vi "PhotonPipelineResult_Equals.vi"(9 "Other PhotonPipelineResult":T1 {"Targets"."CameraToTarget"."ROTATION"."SIN" format="%13.4f"; "Targets"."CameraToTarget"."ROTATION"."COS" format="%13.4f"; "Targets"."CameraToTarget"."ROTATION"."VALUE" format="%13.4f"; "Targets"."CameraToTarget"."TRANSLATION"."Y" format="%14.3f"; "Targets"."CameraToTarget"."TRANSLATION"."X" format="%14.3f"}, 11 "PhotonPipelineResult":T1 {"Targets"."CameraToTarget"."ROTATION"."SIN" format="%13.4f"; "Targets"."CameraToTarget"."ROTATION"."COS" format="%13.4f"; "Targets"."CameraToTarget"."ROTATION"."VALUE" format="%13.4f"; "Targets"."CameraToTarget"."TRANSLATION"."Y" format="%14.3f"; "Targets"."CameraToTarget"."TRANSLATION"."X" format="%14.3f"}) -> (3 "Equal":bool)   [LabVIEW 2019, in "PhotonVisionLib.lvlib"]
doc: "Determines if two PipelineResults are equal.\n\nInputs:\n - PipelineResult -- PipelineResult cluster.\n - Other PipelineResult -- Other PipelineResult cluster.\n\nOutputs:\n - Equal -- Returns TRUE, if both pipeline results are equal.."
uses:
  PhotonVisionLib.lvlib
  TypeDef/PhotonPipelineResultType.ctl
  TypeDef/PhotonTrackedTargetType.ctl
  TypeDef/TargetCornerType.ctl
  <vilib>/Rock Robotics/WPI/ThirdParty/JAS_Junk/TrajLib/TRANSFORM2D.ctl
  <vilib>/Rock Robotics/WPI/ThirdParty/JAS_Junk/TrajLib/TRANSLATION2D.ctl
  <vilib>/Rock Robotics/WPI/ThirdParty/JAS_Junk/TrajLib/ROTATION2D.ctl
  <vilib>/Rock Robotics/WPI/ThirdParty/JAS_Junk/TrajLib/Trajectory_Library.lvlib
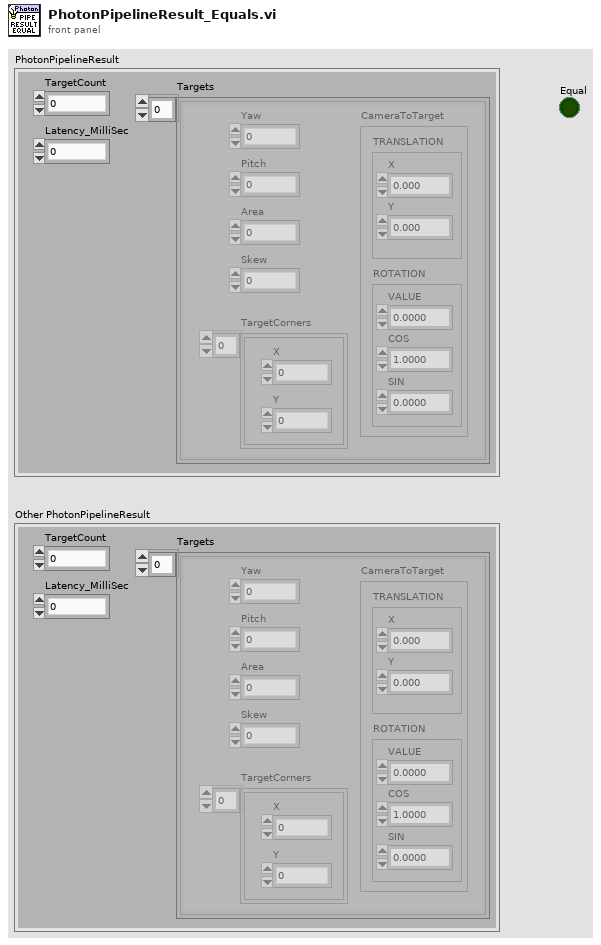
[diagram p1: front panel]
types:
  T1 = typedef "PhotonVisionLib.lvlib/PhotonPipelineResultType.ctl" = cluster{"TargetCount":i32, "Latency_MilliSec":dbl, "Targets":T2[]}
  T2 = typedef "PhotonVisionLib.lvlib/PhotonTrackedTargetType.ctl" = cluster{"Yaw":dbl, "Pitch":dbl, "Area":dbl, "Skew":dbl, "TargetCorners":T3[], "CameraToTarget":T4}
  T3 = typedef "PhotonVisionLib.lvlib/TargetCornerType.ctl" = cluster{"X":dbl, "Y":dbl}
  T4 = typedef "Trajectory_Library.lvlib/TRANSFORM2D.ctl" = cluster{"TRANSLATION":T5, "ROTATION":T6}
  T5 = typedef "Trajectory_Library.lvlib/TRANSLATION2D.ctl" = cluster{"X":dbl, "Y":dbl}
  T6 = typedef "Trajectory_Library.lvlib/ROTATION2D.ctl" = cluster{"VALUE":dbl, "COS":dbl, "SIN":dbl}
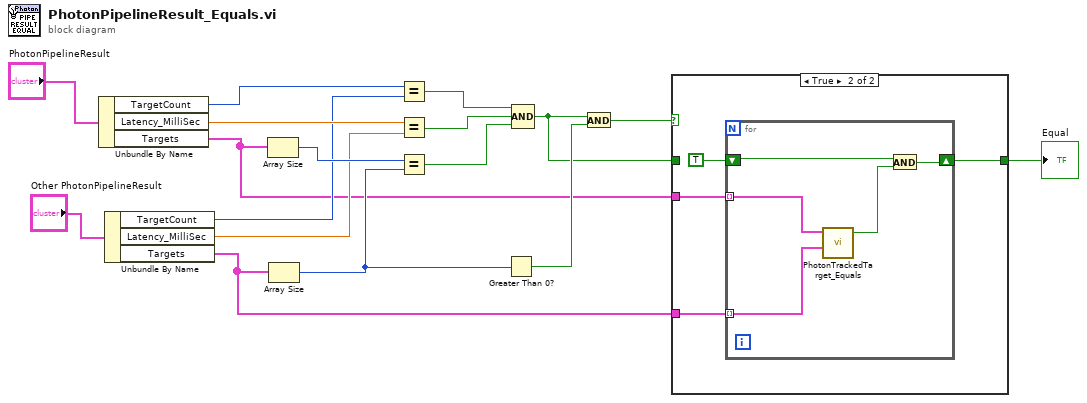
[diagram p0: block diagram]
diagram:
  n1 = Unbundle By Name("PhotonPipelineResult") -> ("TargetCount"=w15:i32, "Latency_MilliSec"=w14:dbl, "Targets"=w4:T2[])
  n2 = Unbundle By Name("Other PhotonPipelineResult") -> ("TargetCount"=w12:i32, "Latency_MilliSec"=w11:dbl, "Targets"=w3:T2[])
  n3 = Array Size(array=w4) -> (size(s)=w13:i32)
  n4 = Array Size(array=w3) -> (size(s)=w7:i32)
  n5 = Equal?(x=w15, y=w12) -> (x = y?=w10:bool)
  n6 = Equal?(x=w14, y=w11) -> (x = y?=w9:bool)
  n7 = Equal?(x=w13, y=w7) -> (x = y?=w8:bool)
  n8 = Greater Than 0?(x=w7) -> (x > 0?=w6:bool)
  n9 = Compound Arithmetic op=AND(w10, w9, w8) -> (w1:bool)
  n10 = And(x=w1, y=w6) -> (x .and. y?=w5:bool)
  n11 = case shown="True" w5 {
    tunnel: w4 -> [_ w22]
    tunnel: w3 -> [_ w21]
    tunnel: [w18 w19] -> w2
    tunnel: w1 -> [w18 _]
    frame False {
    }
    frame True {
      n12 = for {
        tunnel: w22 -> [w27] mode=indexing
        tunnel: w21 -> [w26] mode=indexing
        shift-right: [w25] -> w19
        shift-left: TRUE -> [w24]
        n13 = call "PhotonTrackedTarget_Equals.vi"("Other TrackedTarget"=w26, "TrackedTarget"=w27) -> ("Equals"=w23:bool)  [unwired: 9 in]
        n14 = And(x=w24, y=w23) -> (x .and. y?=w25:bool)
      }
    }
  }
  "Equal" <- w2
